vi "Wait Homing done.vi"(0 "Maximum wait time (sec)":i32=60, 11 "error in (no error)":errorcluster) -> (15 "error out":errorcluster)   [LabVIEW 2024, in "GRBL 1.1.lvlib"]
doc: "Wait till homing procedure is done."
uses:
  GRBL 1.1.lvlib
  Status.ctl
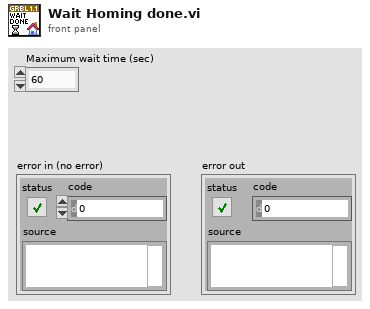
[diagram p1: front panel]
types:
  T1 = typedef "GRBL 1.1.lvlib/Status.ctl" = enum16{"", "Alarm", "Idle", "Run", "Home"}
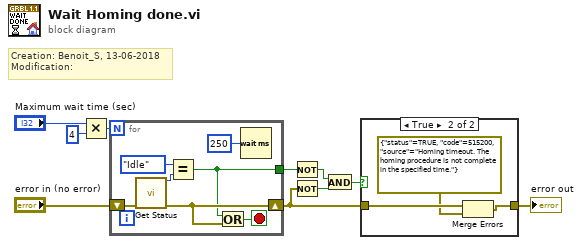
[diagram p0: block diagram]
diagram:
  # "Creation: Benoit_S, 13-06-2018\nModification:"
  n1 = Multiply(x="Maximum wait time (sec)", y=4) -> (x*y=w9:i32)
  n2 = for {
    N: w9 -> [_]
    shift-right: [w14] -> w2
    shift-left: "error in (no error)" -> [w17]
    tunnel: [w11] -> w6
    stop <- w15 stop-if-true
    n3 = call "Get Status.vi"("error in (no error)"=w17) -> ("Status"=w12:T1, "error out"=w14:errorcluster)  [unwired: 10 in, 3 out]
    n4 = Equal?(x=Status."Idle" ("y"), y=w12) -> (x = y?=w11:bool)
    n5 = Or(x=w11, y=w14) -> (x .or. y?=w15:bool)
    n6 = Wait (ms)(milliseconds to wait=u32 250) -> ()  [unwired: 1 out]
  }
  n7 = Not(x=w6) -> (.not. x?=w4:bool)
  n8 = Not(x=w2) -> (.not. x?=w5:bool)
  n9 = And(x=w4, y=w5) -> (x .and. y?=w3:bool)
  n10 = case shown="True" w3 {
    tunnel: w2 -> [w18 w21]
    tunnel: [w18 w19] -> w1
    frame False {
    }
    frame True {
      n11 = Merge Errors(w21, errorcluster {"status"=TRUE, "code"=515200, "source"="Homing timeout. The homing procedure is not complete in the specified time."} ("error constant")) -> (w19:errorcluster)
    }
  }
  "error out" <- w1
